vi "라이센스.vi"() -> ()   [LabVIEW 2014]
panel:
  out "원소":string
  in  "인덱스":i32
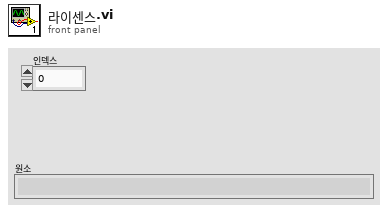
[diagram p1: front panel]
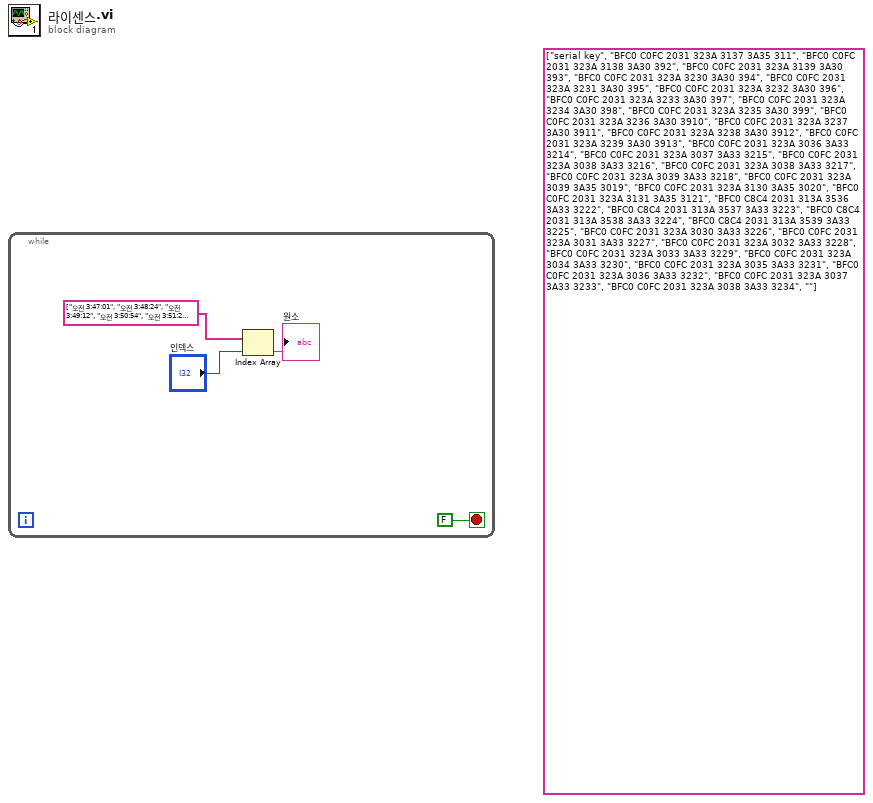
[diagram p0: block diagram]
diagram:
  (unwired) string[] ["serial key", "BFC0 C0FC 2031 323A 3137 3A35 311", "BFC0 C0FC 2031 323A 3138 3A30 392", "BFC0 C0FC 2031 323A 3139 3A30 393", "BFC0 C0FC 2031 323A 3230 3A30 394", "BFC0 C0FC 2031 323A 3231 3A30 395", "BFC0 C0FC 2031 323A 3232 3A30 396", "BFC0 C0FC 2031 323A 3233 3A30 397", "BFC0 C0FC 2031 323A 3234 3A30 398", "BFC0 C0FC 2031 323A 3235 3A30 399", "BFC0 C0FC 2031 323A 3236 3A30 3910", "BFC0 C0FC 2031 323A 3237 3A30 3911", "BFC0 C0FC 2031 323A 3238 3A30 3912", "BFC0 C0FC 2031 323A 3239 3A30 3913", "BFC0 C0FC 2031 323A 3036 3A33 3214", "BFC0 C0FC 2031 323A 3037 3A33 3215", "BFC0 C0FC 2031 323A 3038 3A33 3216", "BFC0 C0FC 2031 323A 3038 3A33 3217", "BFC0 C0FC 2031 323A 3039 3A33 3218", "BFC0 C0FC 2031 323A 3039 3A35 3019", "BFC0 C0FC 2031 323A 3130 3A35 3020", "BFC0 C0FC 2031 323A 3131 3A35 3121", "BFC0 C8C4 2031 313A 3536 3A33 3222", "BFC0 C8C4 2031 313A 3537 3A33 3223", "BFC0 C8C4 2031 313A 3538 3A33 3224", "BFC0 C8C4 2031 313A 3539 3A33 3225", "BFC0 C0FC 2031 323A 3030 3A33 3226", "BFC0 C0FC 2031 323A 3031 3A33 3227", "BFC0 C0FC 2031 323A 3032 3A33 3228", "BFC0 C0FC 2031 323A 3033 3A33 3229", "BFC0 C0FC 2031 323A 3034 3A33 3230", "BFC0 C0FC 2031 323A 3035 3A33 3231", "BFC0 C0FC 2031 323A 3036 3A33 3232", "BFC0 C0FC 2031 323A 3037 3A33 3233", "BFC0 C0FC 2031 323A 3038 3A33 3234", ""] ("출력 배열")
  n1 = while {
    stop <- FALSE stop-if-true
    n2 = Index Array(array=string[] ["오전 3:47:01", "오전 3:48:24", "오전 3:49:12", "오전 3:50:54", "오전 3:51:21", "오전 3:52:33", "오전 3:53:00", "오전 3:54:42", "오전 3:55:41", "오전 3:56:11", "오전 3:57:29", "오전 3:58:59", "오전 3:59:53", "오전 4:00:40"], index="인덱스") -> (element=→"원소":string)
  }
